vi "updateRealTimeInfo.vi"(11 "UI_Data":T1={"controlTabState"=[], "pathToSTLFiles"=path "", "availableObjs"=[], "objectNames"=[], "addedObjs"=[], "selectedObj"={"Name"="", "objectFiles"=[], "center"={"X"=0.0, "Y"=0.0, "Z"=0.0}, "extent"={"X"=0.0, "Y"=0.0, "Z"=0.0}, "allowedMotion"=enum."XY", "mountOn"=enum."yArm", "Movements"=[], "extraInfo"=[], "hasPOI?"=FALSE, "POI"={"X"=0.0, "Y"=0.0, "Z"=0.0}, "posOffset"={"X"=0.0, "Y"=0.0, "Z"=0.0}, "referenceNum"=refnum}, "3DPictureObjRef"=refnum, "yPOI_Home"={"X"=0.0, "Y"=0.0, "Z"=0.0}, "yPOI_Current"={"X"=0.0, "Y"=0.0, "Z"=0.0}, "yPOI_Added?"=FALSE, "homePos_Offset"={"X"=0.0, "Y"=0.0, "Z"=0.0}, "breadBoardOriginOffset"={"X"=0.0, "Y"=0.0, "Z"=0.0}, "XYtranslateObjControls"=[], "ZtranslateObjControls"=[], "pBot_controls"=[], "pBot_VISA"="", "commandLog"="", "pBotConnected?"=FALSE, "pBot_currentEEPROMsettings"="", "realTimeInfoControls"=[], "pBot_tempSensor1"=0.0, "pBot_tempSensor2"=0.0, "realTimeInfoTextColor"=[], "disconnectPBot_Event"=refnum, "needToHomeY?"=FALSE, "pBot_relativePositioning"=FALSE, "pBot_minPos"={"X"=0.0, "Y"=0.0, "Z"=0.0}, "pBot_maxPos"={"X"=0.0, "Y"=0.0, "Z"=0.0}, "pBot_homeOffset"={"X"=0.0, "Y"=0.0, "Z"=0.0}, "textColorGreen"=9174826, "textColorRed"=16750216, "textColorGray"=9868950, "transVisualizationControls"=[], "needToHomeXY?"=FALSE, "pBot_minScanRegion"={"X"=0.0, "Y"=0.0, "Z"=0.0}, "pBot_maxScanRegion"={"X"=0.0, "Y"=0.0, "Z"=0.0}, "pBot_scanN"={"X"=0, "Y"=0, "Z"=0}, "connectedInstruments"=[], "isScanning?"=FALSE, "Wavelengths"=[], "usb2000p_controlRefs"=[]}) -> ()   [LabVIEW 2015]
uses:
  controls/UI Data.ctl
  processedObjectInfo.ctl
  controls/scanInstrumentInfo.ctl
types:
  T1 = typedef "UI Data.ctl" = cluster{"controlTabState":bool[], "pathToSTLFiles":path, "availableObjs":T2[], "objectNames":string[], "addedObjs":T2[], "selectedObj":T2, "3DPictureObjRef":refnum<vi>, "yPOI_Home":cluster{"X":dbl, "Y":dbl, "Z":dbl}, "yPOI_Current":cluster{"X":dbl, "Y":dbl, "Z":dbl}, "yPOI_Added?":bool, "homePos_Offset":cluster{"X":dbl, "Y":dbl, "Z":dbl}, "breadBoardOriginOffset":cluster{"X":dbl, "Y":dbl, "Z":dbl}, "XYtranslateObjControls":refnum<vi>[], "ZtranslateObjControls":refnum<vi>[], "pBot_controls":refnum<vi>[], "pBot_VISA":refnum<visa-resource-name>, "commandLog":string, "pBotConnected?":bool, "pBot_currentEEPROMsettings":string, "realTimeInfoControls":refnum<vi>[], "pBot_tempSensor1":dbl, "pBot_tempSensor2":dbl, "realTimeInfoTextColor":u32[], "disconnectPBot_Event":refnum<user-event>, "needToHomeY?":bool, "pBot_relativePositioning":bool, "pBot_minPos":cluster{"X":dbl, "Y":dbl, "Z":dbl}, "pBot_maxPos":cluster{"X":dbl, "Y":dbl, "Z":dbl}, "pBot_homeOffset":cluster{"X":dbl, "Y":dbl, "Z":dbl}, "textColorGreen":u32, "textColorRed":u32, "textColorGray":u32, "transVisualizationControls":refnum<vi>[], "needToHomeXY?":bool, "pBot_minScanRegion":cluster{"X":sgl, "Y":sgl, "Z":sgl}, "pBot_maxScanRegion":cluster{"X":sgl, "Y":sgl, "Z":sgl}, "pBot_scanN":cluster{"X":u16, "Y":u16, "Z":u16}, "connectedInstruments":T3[], "isScanning?":bool, "Wavelengths":dbl[], "usb2000p_controlRefs":refnum<vi>[]}
  T2 = typedef "processedObjectInfo.ctl" = cluster{"Name":string, "objectFiles":cluster{"Location":path, "Color":cluster{"R":dbl, "G":dbl, "B":dbl, "A":dbl}}[], "center":cluster{"X":dbl, "Y":dbl, "Z":dbl}, "extent":cluster{"X":dbl, "Y":dbl, "Z":dbl}, "allowedMotion":enum16{"XY", "Z"}, "mountOn":enum16{"yArm", "breadBoard"}, "Movements":cluster{"Type":enum16{"rr", "ra", "tr", "ta"}, "vector":cluster{"X":dbl, "Y":dbl, "Z":dbl}, "scalar":dbl}[], "extraInfo":cluster{"parameter":string, "dataType":string, "vector":cluster{"X":dbl, "Y":dbl, "Z":dbl}, "scalar":dbl}[], "hasPOI?":bool, "POI":cluster{"X":dbl, "Y":dbl, "Z":dbl}, "posOffset":cluster{"X":dbl, "Y":dbl, "Z":dbl}, "referenceNum":refnum<vi>}
  T3 = typedef "scanInstrumentInfo.ctl" = cluster{"Name":string, "VISAname":refnum<visa-resource-name>, "1D_dataArraySize":u16, "extraInfo":variant, "error":errorcluster}
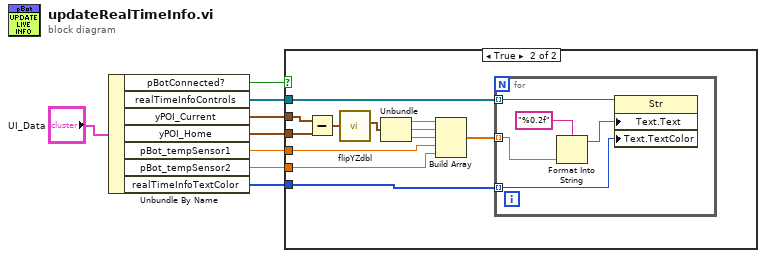
[diagram p0: block diagram]
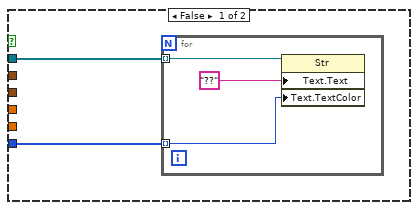
[diagram p2: hidden frame]
diagram:
  n1 = Unbundle By Name("UI_Data") -> ("pBotConnected?"=w2:bool, "realTimeInfoControls"=w3:refnum<vi>[], "yPOI_Current"=w7:cluster{"X":dbl, "Y":dbl, "Z":dbl}, "yPOI_Home"=w6:cluster{"X":dbl, "Y":dbl, "Z":dbl}, "pBot_tempSensor1"=w5:dbl, "pBot_tempSensor2"=w4:dbl, "realTimeInfoTextColor"=w1:u32[])
  n2 = case shown="True" w2 {
    tunnel: w7 -> [_ w25]
    tunnel: w6 -> [_ w24]
    tunnel: w5 -> [_ w20]
    tunnel: w4 -> [_ w19]
    tunnel: w3 -> [w10 w18]
    tunnel: w1 -> [w9 w16]
    frame False {
      n3 = for {
        tunnel: w10 -> [w13] mode=indexing
        tunnel: w9 -> [w12] mode=indexing
        n4 = property class="Str"(reference=w13, "Text.Text"="??" ("format string"), "Text.TextColor"=w12) -> ()  [unwired: 1 in, 2 out]
      }
    }
    frame True {
      n5 = Subtract(x=w25, y=w24) -> (x-y=w15:cluster{"X":dbl, "Y":dbl, "Z":dbl})
      n6 = call "flipYZdbl.vi"("pointIn"=w15) -> ("pointOut"=w14:cluster{"X":dbl, "Y":dbl, "Z":dbl})  [unwired: 10 in]
      n7 = Unbundle(w14) -> ("X"=w23:dbl, "Y"=w22:dbl, "Z"=w21:dbl)
      n8 = Build Array(w23, w22, w21, w20, w19) -> (w17:dbl[])
      n9 = for {
        tunnel: w18 -> [w30] mode=indexing
        tunnel: w17 -> [w28] mode=indexing
        tunnel: w16 -> [w26] mode=indexing
        n10 = Format Into String(format string="%0.2f", w28) -> (resulting string=w27:string)  [unwired: 2 in, 1 out]
        n11 = property class="Str"(reference=w30, "Text.Text"=w27, "Text.TextColor"=w26) -> ()  [unwired: 1 in, 2 out]
      }
    }
  }
